vi "calcOddOrEven.vi"(11 "number":u16) -> (2 "outputNum":u16, 3 "IsEven?":bool)   [LabVIEW 2016]
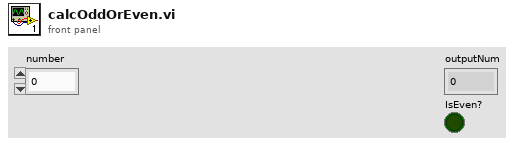
[diagram p1: front panel]
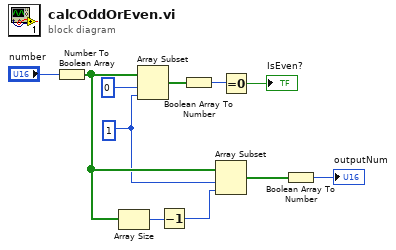
[diagram p0: block diagram]
diagram:
  w7 = 1 ("length")
  n1 = Number To Boolean Array(number="number") -> (Boolean array=w8:bool[])
  n2 = Array Size(array=w8) -> (size(s)=w6:i32)
  n3 = Array Subset(array=w8, index=0, length=w7) -> (w3:bool[])
  n4 = Decrement(x=w6) -> (x-1=w5:i32)
  n5 = Boolean Array To Number(Boolean array=w3) -> (number=w2:u8)
  n6 = Array Subset(array=w8, index=w7, length=w5) -> (w4:bool[])
  n7 = Equal To 0?(x=w2) -> (x = 0?=→"IsEven?":bool)
  n8 = Boolean Array To Number(Boolean array=w4) -> (number=→"outputNum":u16)
